vi "Configure Marker Polarity.vi"(6 "Marker Polarity (0: Positive)":u16(ring) items=["Positive", "Negative"], 8 "error in (no error)":errorcluster, 9 "Marker (0: Marker 1)":u16(ring) items=["Marker1", "Marker2", "Marker3", "Marker4"], 10 "Modulation Format (1: Dual Modulation)":u16(ring)=1 items=["Dual Modulation"=1, "Dual ARB"=2, "Multitone"=3, "Two-tone"=6, "AWGN ARB"=8], 11 "VISA resource name":refnum<visa-resource-name>) -> (0 "error out":errorcluster, 3 "VISA resource name out":refnum<visa-resource-name>)   [LabVIEW 2018, in "Agilent PSG MXG Series.lvlib"]
doc: "Configures the polarity for the marker.\n\n<B>Notes:</B>\n(1) This VI is valid only in E8267C, E8257D, E8267D, N5162A, N5182A, N5172B, N5182B.\n\n(2) For E8267C, this VI is valid only when the instrument installs <B>Option 002</B> (Internal baseband generator) or <B>Option 602</B> (Digital bus baseband generator).\n\n(3) For E8267D, this VI is valid only when the instrument installs <B>Option 601</B> or <B>Option 602</B> (Internal baseband generator).\n\n(4) For N5162A and N5182A, this VI is valid only when the instrument installs <B>Option 651</B> or <B>Option 652</B> or <B>Option 654</B> (Internal baseband generator)."
uses:
  Agilent PSG MXG Series.lvlib
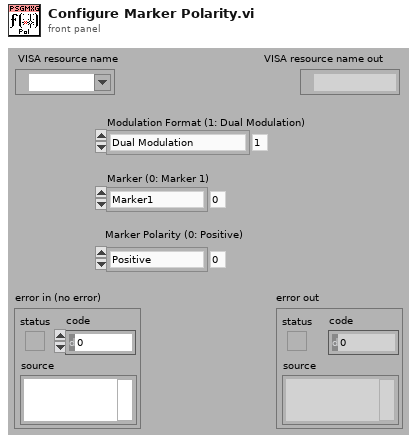
[diagram p1: front panel]
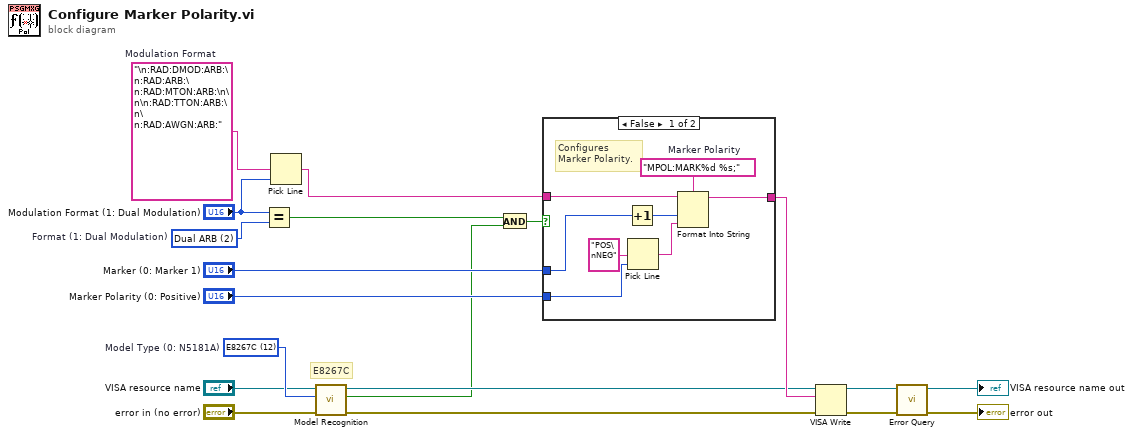
[diagram p0: block diagram]
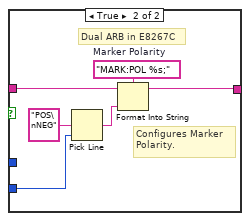
[diagram p2: hidden frame]
diagram:
  w6 = u16 12 items=["N5181A"=0, "N5182A"=1, "E8241A"=5, "E8244A"=6, "E8251A"=7, "E8254A"=8, "E8247C"=10, "E8257C"=11, "E8267C"=12, "E8257D"=15, "E8267D"=16]  # Model Type (0: N5181A)
  w17 = u16 2 items=["Dual Modulation"=1, "Dual ARB"=2]  # Format (1: Dual Modulation)
  w19 = "\n:RAD:DMOD:ARB:\n:RAD:ARB:\n:RAD:MTON:ARB:\n\n\n:RAD:TTON:ARB:\n\n:RAD:AWGN:ARB:"  # Modulation Format
  # "E8267C"
  n1 = Equal?(x="Modulation Format (1: Dual Modulation)", y=w17) -> (x = y?=w16:bool)
  n2 = Pick Line(multi-line string=w19, line index="Modulation Format (1: Dual Modulation)") -> (output string=w14:string)  [unwired: 1 out]
  n3 = call "Model Recognition.vi"("error in (no error)"="error in (no error)", "Model Type (0: N5181A)"=w6, "VISA resource name"="VISA resource name") -> ("error out"=w7:errorcluster, "Is Model Correct"=w5:bool, "VISA resource name out"=w8:refnum<visa-resource-name>)  [unwired: 6 out]
  n4 = And(x=w16, y=w5) -> (x .and. y?=w15:bool)
  n5 = case shown="False" w15 {
    tunnel: w14 -> [w26 w32]
    tunnel: "Marker Polarity (0: Positive)" -> [w23 w29]
    tunnel: "Marker (0: Marker 1)" -> [w20 _]
    tunnel: [w22 w28] -> w11
    frame False {
      w27 = "MPOL:MARK%d %s;"  # Marker Polarity
      # "Configures\nMarker Polarity."
      n6 = Increment(x=w20) -> (x+1=w21:u16)
      n7 = Pick Line(multi-line string="POS\nNEG", line index=w23) -> (output string=w24:string)  [unwired: 1 out]
      n8 = Format Into String(format string=w27, initial string=w26, w21, w24) -> (resulting string=w22:string)  [unwired: 1 in, 1 out]
    }
    frame True {
      w33 = "MARK:POL %s;"  # Marker Polarity
      # "Configures Marker\nPolarity."
      # "Dual ARB in E8267C"
      n9 = Pick Line(multi-line string="POS\nNEG", line index=w29) -> (output string=w31:string)  [unwired: 1 out]
      n10 = Format Into String(format string=w33, initial string=w32, w31) -> (resulting string=w28:string)  [unwired: 1 in, 1 out]
    }
  }
  n11 = VISA Write(VISA resource name=w8, write buffer=w11, error in (no error)=w7) -> (VISA resource name out=w10:refnum<visa-resource-name>, error out=w9:errorcluster)  [unwired: 1 out]
  n12 = call "Error Query.vi"("error in (no error)"=w9, "VISA resource name"=w10) -> ("error out"=→"error out":errorcluster, "VISA resource name out"=→"VISA resource name out":refnum<visa-resource-name>)  [unwired: 8 out]
